vi "enumerateStaticDependencies.vi"(8 "error in (no error)":errorcluster, 11 "Instrument":refnum<class "Instrument.lvclass">) -> (0 "error out":errorcluster, 2 "Static Dependencies":refnum<class "Dependency.lvclass">[](array[class]), 3 "Instrument out":refnum<class "Instrument.lvclass">)   [LabVIEW 2019, in "Instrument.lvclass"]
doc: "JKI State Machine Objects (SMO) 1.3.0.56\nJKI - JKI\nCopyright (c) 2017, JKI"
uses:
  Instrument.lvclass
  C:/Program Files (x86)/National Instruments/LabVIEW 2019/vi.lib/JKI/JKI SMO/SMO/SMO.lvclass
  <vilib>/JKI/JKI SMO/Dependency/Dependency.lvclass
  <userlib>/LevyLab/Logger.Error/Logger.Error.lvclass
  C:/Program Files (x86)/National Instruments/LabVIEW 2019/user.lib/LevyLab/Logger/Logger.lvclass
  <userlib>/LevyLab/Logger.PGSQL/Logger.PGSQL.lvclass
  <userlib>/LevyLab/Logger.Error/Logger.Error.lvclass/Logger.Error.ctl
  <userlib>/LevyLab/RemoteControl/RemoteControl.lvclass
  subsystems/HAL/HAL.lvclass
  <vilib>/JKI/JKI SMO/SMO/SMO.lvclass
  <userlib>/LevyLab/Logger/Logger.lvclass
panel:
  # "For instructions on how to use the JKI State Machine Objects, examples and video tutorials, visit:\nhttp://jki.net/state-machine-objects/\n\nJKI State Machine Objects™\nhttp://jki.net/state-machine-objects/\nCopyright (C) 2005-2015, JKI <info@jki.net>\nALL RIGHTS RESERVED"
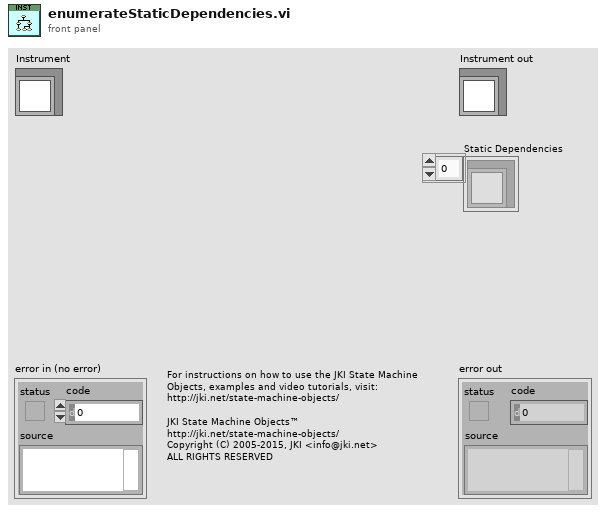
[diagram p1: front panel]
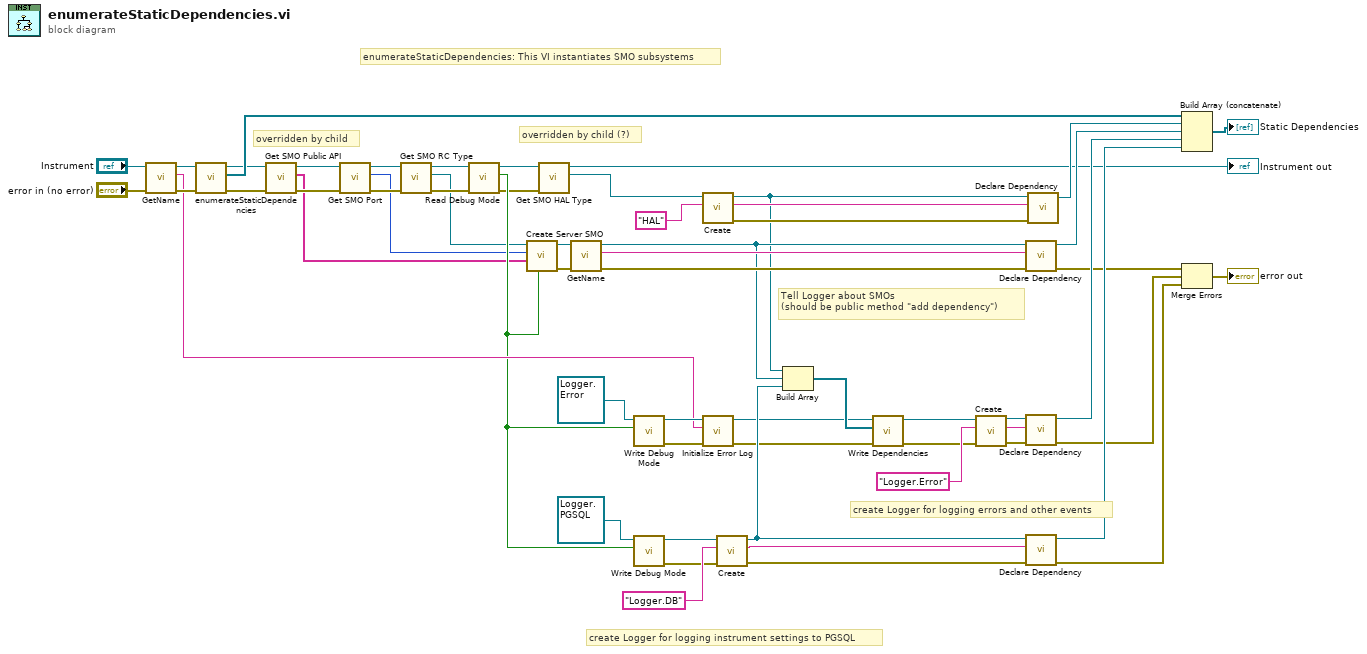
[diagram p0: block diagram]
diagram:
  # "overridden by child (?)"
  # "enumerateStaticDependencies: This VI instantiates SMO subsystems"
  # "Tell Logger about SMOs\n(should be public method \"add dependency\")"
  # "create Logger for logging errors and other events"
  # "create Logger for logging instrument settings to PGSQL"
  # "overridden by child"
  n1 = call <vilib>:"GetName.vi"("error in (no error)"="error in (no error)", "SMO"="Instrument") -> ("error out"=w55:errorcluster, "Name"=w21:string, "SMO out"=w56:refnum<class "Instrument.lvclass">)  [unwired: 6 in, 1 out]
  n2 = call-parent "enumerateStaticDependencies.vi"("error in (no error)"=w55, "SMO"=w56) -> ("error out"=w17:errorcluster, "Static Dependencies"=w30:refnum<class "Dependency.lvclass">[], "SMO out"=w18:refnum<class "Instrument.lvclass">)  [unwired: 7 in]
  n3 = call-dynamic "Get SMO Public API.vi"("error in (no error)"=w17, "Instrument in"=w18) -> ("error out"=w19:errorcluster, "commands"=w1:string[], "Instrument out"=w43:refnum<class "Instrument.lvclass">)  [unwired: 7 in]
  n4 = call-dynamic "Get SMO Port.vi"("error in (no error)"=w19, "Instrument in"=w43) -> ("error out"=w15:errorcluster, "Port"=w12:u16, "Instrument out"=w16:refnum<class "Instrument.lvclass">)  [unwired: 7 in]
  n5 = call-dynamic "Get SMO RC Type.vi"("error in (no error)"=w15, "Instrument in"=w16) -> ("error out"=w14:errorcluster, "RemoteControl"=w11:refnum<class "RemoteControl.lvclass">, "Instrument out"=w13:refnum<class "Instrument.lvclass">)  [unwired: 7 in]
  n6 = call-dynamic "Read Debug Mode.vi"("error in (no error)"=w14, "Instrument in"=w13) -> ("error out"=w2:errorcluster, "Debug Mode?"=w20:bool, "Instrument out"=w9:refnum<class "Instrument.lvclass">)  [unwired: 7 in]
  n7 = call <userlib>:"Create Server SMO.vi"("Debug Mode?"=w20, "Commands"=w1, "Port"=w12, "RemoteControl in"=w11) -> ("error out"=w32:errorcluster, "RemoteControl out"=w33:refnum<class "RemoteControl.lvclass">)  [unwired: 6 in]
  n8 = call-dynamic "Get SMO HAL Type.vi"("error in (no error)"=w2, "Instrument in"=w9) -> ("Dependencies.HAL"=w7:refnum<class "HAL.lvclass">, "Instrument out"=→"Instrument out":refnum<class "Instrument.lvclass">)  [unwired: 7 in, 1 out]
  n9 = call <vilib>:"GetName.vi"("error in (no error)"=w32, "SMO"=w33) -> ("error out"=w35:errorcluster, "Name"=w36:string, "SMO out"=w29:refnum<class "RemoteControl.lvclass">)  [unwired: 6 in, 1 out]
  n10 = call <userlib>:"Write Debug Mode.vi"("Debug Mode?"=w20, "Logger in"=refnum<class "Logger.Error.lvclass"> refnum ("Logger.Error.lvclass")) -> ("error out"=w25:errorcluster, "Logger out"=w24:refnum<class "Logger.Error.lvclass">)  [unwired: 8 in]
  n11 = call <userlib>:"Write Debug Mode.vi"("Debug Mode?"=w20, "Logger in"=refnum<class "Logger.PGSQL.lvclass"> refnum ("Logger.PGSQL.lvclass")) -> ("error out"=w46:errorcluster, "Logger out"=w45:refnum<class "Logger.PGSQL.lvclass">)  [unwired: 8 in]
  n12 = call <vilib>:"Create.vi"("Subsystem Name (optional)"="HAL" ("Name"), "SMO"=w7) -> ("error out"=w6:errorcluster, "SMO name"=w5:string, "SMO out"=w3:refnum<class "HAL.lvclass">)  [unwired: 7 in]
  n13 = call <userlib>:"Initialize Error Log.vi"("error in (no error)"=w25, "Application Name"=w21, "Logger.Error in"=w24) -> ("error out"=w22:errorcluster, "Logger.Error out"=w23:refnum<class "Logger.Error.lvclass">)  [unwired: 7 in]
  n14 = call <vilib>:"Create.vi"("error in (no error)"=w46, "Subsystem Name (optional)"="Logger.DB" ("Name"), "SMO"=w45) -> ("error out"=w48:errorcluster, "SMO name"=w26:string, "SMO out"=w38:refnum<class "Logger.PGSQL.lvclass">)  [unwired: 6 in]
  n15 = Build Array(w3, w29, w38) -> (w37:refnum<class "SMO.lvclass">[])
  n16 = call <userlib>:"Write Dependencies.vi"("error in (no error)"=w22, "SMOs"=w37, "Logger.Error in"=w23) -> ("error out"=w39:errorcluster, "Logger.Error out"=w40:refnum<class "Logger.Error.lvclass">)  [unwired: 7 in]
  n17 = call <vilib>:"Create.vi"("error in (no error)"=w39, "Subsystem Name (optional)"="Logger.Error" ("Name"), "SMO"=w40) -> ("error out"=w50:errorcluster, "SMO name"=w27:string, "SMO out"=w51:refnum<class "Logger.Error.lvclass">)  [unwired: 6 in]
  n18 = call <vilib>:"Declare Dependency.vi"("error in (no error)"=w35, "Name"=w36, "Type"=w29) -> ("error out"=w34:errorcluster, "Dependency out"=w41:refnum<class "Dependency.lvclass">)  [unwired: 7 in]
  n19 = call <vilib>:"Declare Dependency.vi"("error in (no error)"=w50, "Name"=w27, "Type"=w51) -> ("error out"=w31:errorcluster, "Dependency out"=w53:refnum<class "Dependency.lvclass">)  [unwired: 7 in]
  n20 = call <vilib>:"Declare Dependency.vi"("error in (no error)"=w48, "Name"=w26, "Type"=w38) -> ("error out"=w42:errorcluster, "Dependency out"=w44:refnum<class "Dependency.lvclass">)  [unwired: 7 in]
  n21 = call <vilib>:"Declare Dependency.vi"("error in (no error)"=w6, "Name"=w5, "Type"=w3) -> ("Dependency out"=w10:refnum<class "Dependency.lvclass">)  [unwired: 7 in, 1 out]
  n22 = Build Array (concatenate)(w30, w10, w41, w53, w44) -> (→"Static Dependencies":refnum<class "Dependency.lvclass">[])
  n23 = Merge Errors(w34, w31, w42) -> (→"error out":errorcluster)
